vi "Cycling_No_DAQ_Tasks_All_3_PS.vi"() -> ()   [LabVIEW 2020]
uses:
  Desktop/Battery-Testing-Software - Shortcut.lnk/Drivers-IT-M3400/IT-M3400.lvlib
panel:
  in  "Number of Cycles 3":i32
  in  "Charge filepath 3":path
  in  "Discharge filepath 3":path
  in  "Batteryname 3":string
  in  "Starting Cycle 3":i32
  out "PS Visa Out 3":refnum<visa-resource-name>
  out "PS error out 3":errorcluster
  in  "Wait time 3":dbl
  in  "Discharge Current Setpoint 3":dbl format="%#.6g"
  in  "Charge Current Setpoint 3":dbl format="%#.6g"
  in  "Battery Type 3":enum16{"30Q", "40T"}(ring)
  in  "PS type 3":enum16{"NHR", "ITECH"}(ring)
  in  "PS error in 3":errorcluster caption="PS error in (no error)"
  in  "PS VISA in 3":refnum<visa-resource-name>
  in  "Number of Cycles 2":i32
  in  "Charge filepath 2":path
  in  "Discharge filepath 2":path
  in  "Batteryname 2":string
  in  "Starting Cycle 2":i32
  out "PS Visa Out 2":refnum<visa-resource-name>
  out "PS error out 2":errorcluster
  in  "Wait time 2":dbl
  in  "Discharge Current Setpoint 2":dbl format="%#.6g"
  in  "Charge Current Setpoint 2":dbl format="%#.6g"
  in  "Battery Type 2":enum16{"30Q", "40T"}(ring)
  in  "PS type 2":enum16{"NHR", "ITECH"}(ring)
  in  "PS error in 2":errorcluster caption="PS error in (no error)"
  in  "PS VISA in 2":refnum<visa-resource-name>
  in  "Number of Cycles":i32
  in  "Charge filepath":path
  in  "Discharge filepath":path
  in  "Batteryname":string
  in  "Starting Cycle":i32
  out "PS error out":errorcluster
  out "PS Visa Out":refnum<visa-resource-name>
  in  "Wait time":dbl
  in  "Discharge Current Setpoint":dbl format="%#.6g"
  in  "Charge Current Setpoint":dbl format="%#.6g"
  in  "Battery Type":enum16{"30Q", "40T"}(ring)
  in  "PS type":enum16{"NHR", "ITECH"}(ring)
  in  "PS error in":errorcluster caption="PS error in (no error)"
  in  "PS VISA in":refnum<visa-resource-name>
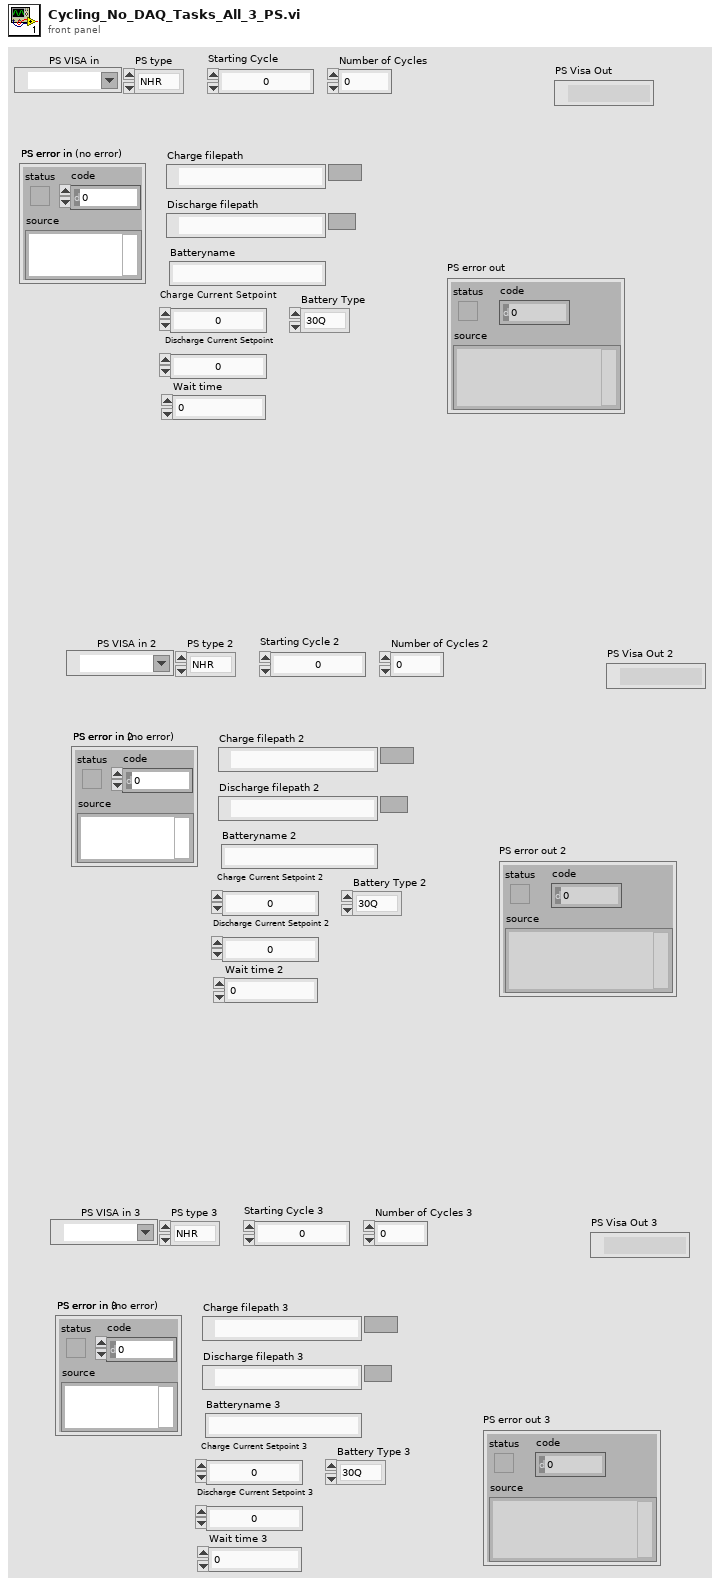
[diagram p1: front panel]
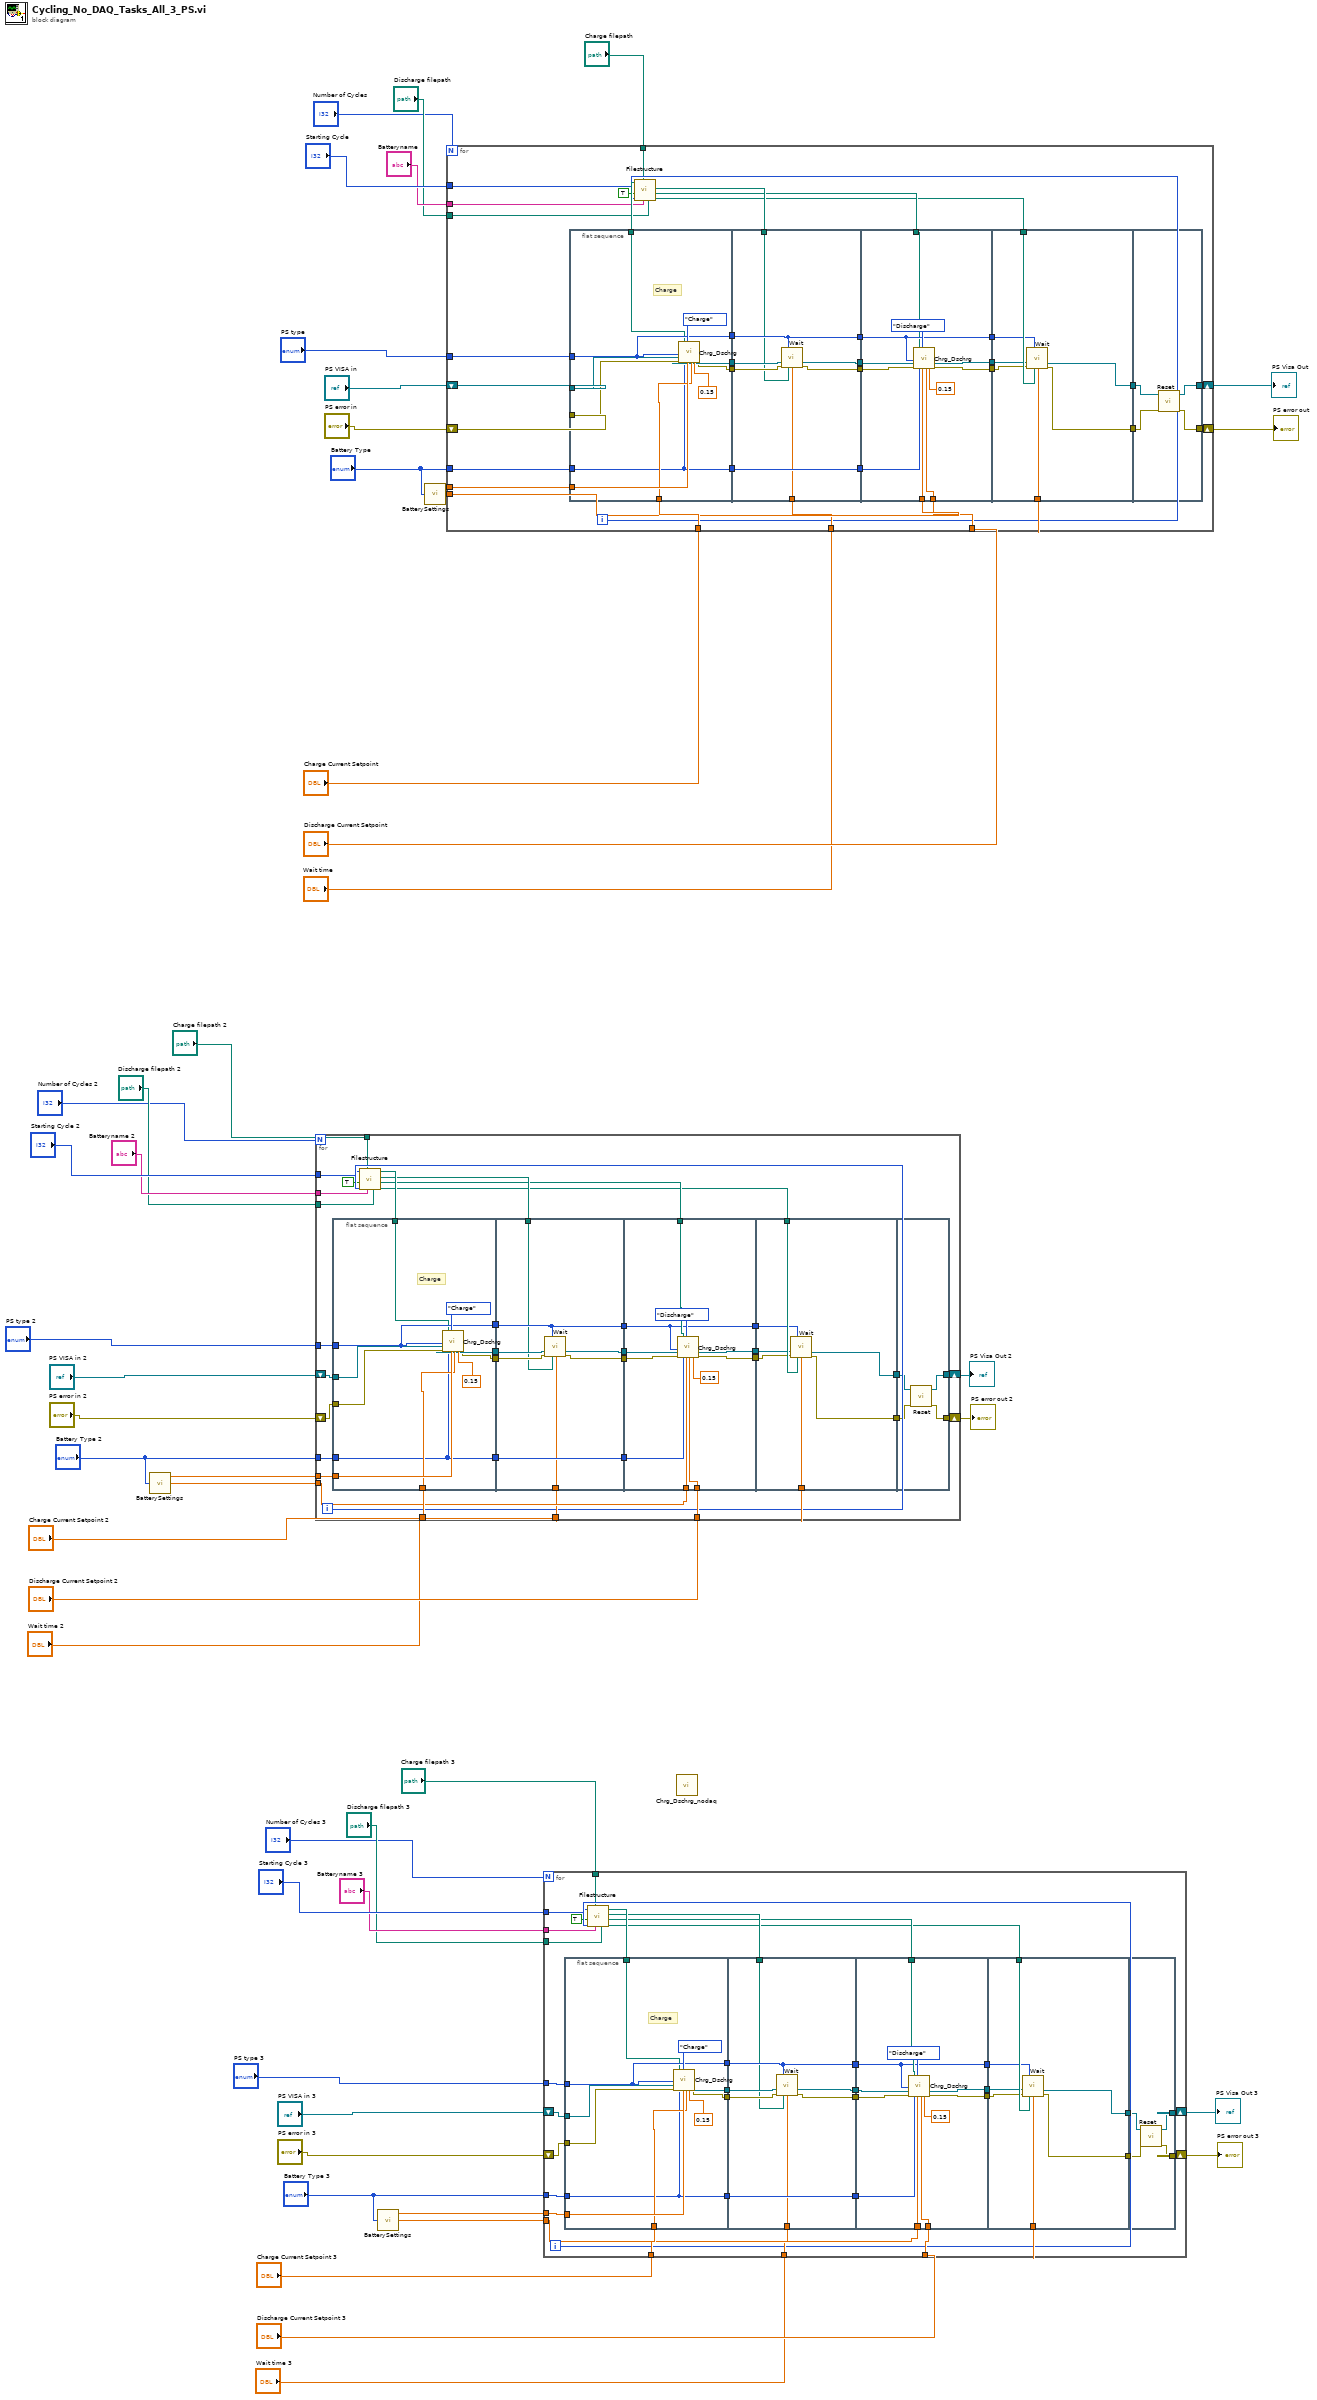
[diagram p0: block diagram]
diagram:
  n1 = call "BatterySettings.vi"("Battery Type"="Battery Type 2") -> ("Min Voltage (V)"=w26:dbl, "Max Voltage (V)"=w29:dbl)  [unwired: 2 in, 1 out]
  n2 = for {
    N: "Number of Cycles 2" -> [_]
    tunnel: "PS type 2" -> [w71]
    tunnel: w29 -> [w68]
    tunnel: "Battery Type 2" -> [w67]
    tunnel: "Charge Current Setpoint 2" -> [w66]
    tunnel: w26 -> [w65]
    tunnel: "Discharge Current Setpoint 2" -> [w64]
    tunnel: "Wait time 2" -> [w59]
    shift-right: [w57] -> w22
    shift-left: "PS VISA in 2" -> [w70]
    shift-right: [w58] -> w23
    shift-left: "PS error in 2" -> [w69]
    tunnel: "Starting Cycle 2" -> [w55]
    tunnel: "Batteryname 2" -> [w53]
    tunnel: "Discharge filepath 2" -> [w52]
    tunnel: "Charge filepath 2" -> [w51]
    i -> [w56]
    n3 = flat-sequence {
      tunnel: w71 -> [w85]
      tunnel: w70 -> [w93]
      tunnel: w69 -> [w92]
      tunnel: w67 -> [w84]
      tunnel: w68 -> [w89]
      tunnel: w66 -> [w88]
      tunnel: [w87] -> w82
      tunnel: [w86] -> w81
      tunnel: [w85] -> w80
      tunnel: [w84] -> w79
      tunnel: w63 -> [w83]
      tunnel: w82 -> [w101]
      tunnel: w81 -> [w100]
      tunnel: w80 -> [w97]
      tunnel: [w99] -> w78
      tunnel: [w98] -> w77
      tunnel: [w97] -> w76
      tunnel: w79 -> [w96]
      tunnel: [w96] -> w75
      tunnel: w62 -> [w95]
      tunnel: w59 -> [w94]
      tunnel: w78 -> [w112]
      tunnel: w77 -> [w111]
      tunnel: w76 -> [w102]
      tunnel: w75 -> [w110]
      tunnel: w65 -> [w109]
      tunnel: w64 -> [w108]
      tunnel: w61 -> [w105]
      tunnel: [w104] -> w74
      tunnel: [w103] -> w73
      tunnel: [w102] -> w72
      tunnel: w60 -> [w119]
      tunnel: w74 -> [w118]
      tunnel: w73 -> [w117]
      tunnel: w59 -> [w116]
      tunnel: w72 -> [w115]
      tunnel: [w114] -> w50
      tunnel: [w113] -> w49
      tunnel: [w122] -> w57
      tunnel: [w120] -> w58
      tunnel: w50 -> [w121]
      tunnel: w49 -> [w123]
      frame #0 {
        # "Charge"
        n4 = call "Chrg_Dschrg.vi"("PS type"=w85, "PS VISA in"=w93, "PS error in"=w92, "DischargeCyclePath"=w83, "Battery Type"=w84, "Charge/discharge"=enum8{"Charge", "Discharge"}."Charge", "Charge/Discharge Voltage Setpoint"=w89, "Current Setpoint"=w88, "Current Cutoff"=0.15) -> ("PS VIS resource name out"=w87:refnum<visa-resource-name>, "PS error out"=w86:errorcluster)  [unwired: 7 in, 2 out]
      }
      frame #1 {
        n5 = call "Wait.vi"("PS type"=w97, "PS VISA in"=w101, "PS error in"=w100, "Wait Filepath"=w95, "Wait time"=w94) -> ("PS Visa Out"=w99:refnum<visa-resource-name>, "PS error out"=w98:errorcluster)  [unwired: 7 in, 2 out]
      }
      frame #2 {
        n6 = call "Chrg_Dschrg.vi"("PS type"=w102, "PS VISA in"=w112, "PS error in"=w111, "DischargeCyclePath"=w105, "Battery Type"=w110, "Charge/discharge"=enum8{"Charge", "Discharge"}."Discharge", "Charge/Discharge Voltage Setpoint"=w109, "Current Setpoint"=w108, "Current Cutoff"=0.15) -> ("PS VIS resource name out"=w104:refnum<visa-resource-name>, "PS error out"=w103:errorcluster)  [unwired: 7 in, 2 out]
      }
      frame #3 {
        n7 = call "Wait.vi"("PS type"=w115, "PS VISA in"=w118, "PS error in"=w117, "Wait Filepath"=w119, "Wait time"=w116) -> ("PS Visa Out"=w113:refnum<visa-resource-name>, "PS error out"=w114:errorcluster)  [unwired: 7 in, 2 out]
      }
      frame #4 {
        n8 = call "Reset.vi"("error in"=w121, "VISA resource name"=w123) -> ("error out"=w120:errorcluster, "VISA resource name out"=w122:refnum<visa-resource-name>)  [unwired: 8 in]
      }
    }
    n9 = call "Filestructure.vi"("Discharge filepath"=w52, "Batteryname"=w53, "Charge filepath"=w51, "For loop i"=w56, "In for loop"=TRUE, "Starting Cycle"=w55) -> ("DischargeWaitPath"=w60:path, "DischargeCyclePath"=w61:path, "ChargeWaitPath"=w62:path, "ChargeCyclePath"=w63:path)  [unwired: 1 in, 1 out]
  }
  "PS error out 2" <- w23
  "PS Visa Out 2" <- w22
  n10 = call "BatterySettings.vi"("Battery Type"="Battery Type 3") -> ("Min Voltage (V)"=w10:dbl, "Max Voltage (V)"=w13:dbl)  [unwired: 2 in, 1 out]
  n11 = call "BatterySettings.vi"("Battery Type"="Battery Type") -> ("Min Voltage (V)"=w42:dbl, "Max Voltage (V)"=w45:dbl)  [unwired: 2 in, 1 out]
  n12 = for {
    N: "Number of Cycles" -> [_]
    tunnel: "PS type" -> [w146]
    tunnel: w45 -> [w143]
    tunnel: "Battery Type" -> [w142]
    tunnel: "Charge Current Setpoint" -> [w141]
    tunnel: w42 -> [w140]
    tunnel: "Discharge Current Setpoint" -> [w139]
    tunnel: "Wait time" -> [w134]
    shift-right: [w132] -> w38
    shift-left: "PS VISA in" -> [w145]
    shift-right: [w133] -> w39
    shift-left: "PS error in" -> [w144]
    tunnel: "Starting Cycle" -> [w130]
    tunnel: "Batteryname" -> [w128]
    tunnel: "Discharge filepath" -> [w127]
    tunnel: "Charge filepath" -> [w126]
    i -> [w131]
    n13 = flat-sequence {
      tunnel: w146 -> [w160]
      tunnel: w145 -> [w168]
      tunnel: w144 -> [w167]
      tunnel: w142 -> [w159]
      tunnel: w143 -> [w164]
      tunnel: w141 -> [w163]
      tunnel: [w162] -> w157
      tunnel: [w161] -> w156
      tunnel: [w160] -> w155
      tunnel: [w159] -> w154
      tunnel: w138 -> [w158]
      tunnel: w157 -> [w176]
      tunnel: w156 -> [w175]
      tunnel: w155 -> [w172]
      tunnel: [w174] -> w153
      tunnel: [w173] -> w152
      tunnel: [w172] -> w151
      tunnel: w154 -> [w171]
      tunnel: [w171] -> w150
      tunnel: w137 -> [w170]
      tunnel: w134 -> [w169]
      tunnel: w153 -> [w187]
      tunnel: w152 -> [w186]
      tunnel: w151 -> [w178]
      tunnel: w150 -> [w185]
      tunnel: w140 -> [w184]
      tunnel: w139 -> [w183]
      tunnel: w136 -> [w177]
      tunnel: [w180] -> w149
      tunnel: [w179] -> w148
      tunnel: [w178] -> w147
      tunnel: w135 -> [w194]
      tunnel: w149 -> [w193]
      tunnel: w148 -> [w192]
      tunnel: w134 -> [w191]
      tunnel: w147 -> [w190]
      tunnel: [w189] -> w125
      tunnel: [w188] -> w124
      tunnel: [w197] -> w132
      tunnel: [w195] -> w133
      tunnel: w125 -> [w196]
      tunnel: w124 -> [w198]
      frame #0 {
        # "Charge"
        n14 = call "Chrg_Dschrg.vi"("PS type"=w160, "PS VISA in"=w168, "PS error in"=w167, "DischargeCyclePath"=w158, "Battery Type"=w159, "Charge/discharge"=enum8{"Charge", "Discharge"}."Charge", "Charge/Discharge Voltage Setpoint"=w164, "Current Setpoint"=w163, "Current Cutoff"=0.15) -> ("PS VIS resource name out"=w162:refnum<visa-resource-name>, "PS error out"=w161:errorcluster)  [unwired: 7 in, 2 out]
      }
      frame #1 {
        n15 = call "Wait.vi"("PS type"=w172, "PS VISA in"=w176, "PS error in"=w175, "Wait Filepath"=w170, "Wait time"=w169) -> ("PS Visa Out"=w174:refnum<visa-resource-name>, "PS error out"=w173:errorcluster)  [unwired: 7 in, 2 out]
      }
      frame #2 {
        n16 = call "Chrg_Dschrg.vi"("PS type"=w178, "PS VISA in"=w187, "PS error in"=w186, "DischargeCyclePath"=w177, "Battery Type"=w185, "Charge/discharge"=enum8{"Charge", "Discharge"}."Discharge", "Charge/Discharge Voltage Setpoint"=w184, "Current Setpoint"=w183, "Current Cutoff"=0.15) -> ("PS VIS resource name out"=w180:refnum<visa-resource-name>, "PS error out"=w179:errorcluster)  [unwired: 7 in, 2 out]
      }
      frame #3 {
        n17 = call "Wait.vi"("PS type"=w190, "PS VISA in"=w193, "PS error in"=w192, "Wait Filepath"=w194, "Wait time"=w191) -> ("PS Visa Out"=w188:refnum<visa-resource-name>, "PS error out"=w189:errorcluster)  [unwired: 7 in, 2 out]
      }
      frame #4 {
        n18 = call "Reset.vi"("error in"=w196, "VISA resource name"=w198) -> ("error out"=w195:errorcluster, "VISA resource name out"=w197:refnum<visa-resource-name>)  [unwired: 8 in]
      }
    }
    n19 = call "Filestructure.vi"("Discharge filepath"=w127, "Batteryname"=w128, "Charge filepath"=w126, "For loop i"=w131, "In for loop"=TRUE, "Starting Cycle"=w130) -> ("DischargeWaitPath"=w135:path, "DischargeCyclePath"=w136:path, "ChargeWaitPath"=w137:path, "ChargeCyclePath"=w138:path)  [unwired: 1 in, 1 out]
  }
  "PS error out" <- w39
  "PS Visa Out" <- w38
  n20 = for {
    N: "Number of Cycles 3" -> [_]
    tunnel: "PS type 3" -> [w221]
    tunnel: w13 -> [w218]
    tunnel: "Battery Type 3" -> [w217]
    tunnel: "Charge Current Setpoint 3" -> [w216]
    tunnel: w10 -> [w215]
    tunnel: "Discharge Current Setpoint 3" -> [w214]
    tunnel: "Wait time 3" -> [w209]
    shift-right: [w207] -> w6
    shift-left: "PS VISA in 3" -> [w220]
    shift-right: [w208] -> w7
    shift-left: "PS error in 3" -> [w219]
    tunnel: "Starting Cycle 3" -> [w205]
    tunnel: "Batteryname 3" -> [w203]
    tunnel: "Discharge filepath 3" -> [w202]
    tunnel: "Charge filepath 3" -> [w201]
    i -> [w206]
    n21 = flat-sequence {
      tunnel: w221 -> [w235]
      tunnel: w220 -> [w243]
      tunnel: w219 -> [w242]
      tunnel: w217 -> [w234]
      tunnel: w218 -> [w239]
      tunnel: w216 -> [w238]
      tunnel: [w237] -> w232
      tunnel: [w236] -> w231
      tunnel: [w235] -> w230
      tunnel: [w234] -> w229
      tunnel: w213 -> [w233]
      tunnel: w232 -> [w251]
      tunnel: w231 -> [w250]
      tunnel: w230 -> [w247]
      tunnel: [w249] -> w228
      tunnel: [w248] -> w227
      tunnel: [w247] -> w226
      tunnel: w229 -> [w246]
      tunnel: [w246] -> w225
      tunnel: w212 -> [w245]
      tunnel: w209 -> [w244]
      tunnel: w228 -> [w262]
      tunnel: w227 -> [w261]
      tunnel: w226 -> [w252]
      tunnel: w225 -> [w260]
      tunnel: w215 -> [w259]
      tunnel: w214 -> [w258]
      tunnel: w211 -> [w255]
      tunnel: [w254] -> w224
      tunnel: [w253] -> w223
      tunnel: [w252] -> w222
      tunnel: w210 -> [w269]
      tunnel: w224 -> [w268]
      tunnel: w223 -> [w267]
      tunnel: w209 -> [w266]
      tunnel: w222 -> [w265]
      tunnel: [w264] -> w200
      tunnel: [w263] -> w199
      tunnel: [w272] -> w207
      tunnel: [w270] -> w208
      tunnel: w200 -> [w271]
      tunnel: w199 -> [w273]
      frame #0 {
        # "Charge"
        n22 = call "Chrg_Dschrg.vi"("PS type"=w235, "PS VISA in"=w243, "PS error in"=w242, "DischargeCyclePath"=w233, "Battery Type"=w234, "Charge/discharge"=enum8{"Charge", "Discharge"}."Charge", "Charge/Discharge Voltage Setpoint"=w239, "Current Setpoint"=w238, "Current Cutoff"=0.15) -> ("PS VIS resource name out"=w237:refnum<visa-resource-name>, "PS error out"=w236:errorcluster)  [unwired: 7 in, 2 out]
      }
      frame #1 {
        n23 = call "Wait.vi"("PS type"=w247, "PS VISA in"=w251, "PS error in"=w250, "Wait Filepath"=w245, "Wait time"=w244) -> ("PS Visa Out"=w249:refnum<visa-resource-name>, "PS error out"=w248:errorcluster)  [unwired: 7 in, 2 out]
      }
      frame #2 {
        n24 = call "Chrg_Dschrg.vi"("PS type"=w252, "PS VISA in"=w262, "PS error in"=w261, "DischargeCyclePath"=w255, "Battery Type"=w260, "Charge/discharge"=enum8{"Charge", "Discharge"}."Discharge", "Charge/Discharge Voltage Setpoint"=w259, "Current Setpoint"=w258, "Current Cutoff"=0.15) -> ("PS VIS resource name out"=w254:refnum<visa-resource-name>, "PS error out"=w253:errorcluster)  [unwired: 7 in, 2 out]
      }
      frame #3 {
        n25 = call "Wait.vi"("PS type"=w265, "PS VISA in"=w268, "PS error in"=w267, "Wait Filepath"=w269, "Wait time"=w266) -> ("PS Visa Out"=w263:refnum<visa-resource-name>, "PS error out"=w264:errorcluster)  [unwired: 7 in, 2 out]
      }
      frame #4 {
        n26 = call "Reset.vi"("error in"=w271, "VISA resource name"=w273) -> ("error out"=w270:errorcluster, "VISA resource name out"=w272:refnum<visa-resource-name>)  [unwired: 8 in]
      }
    }
    n27 = call "Filestructure.vi"("Discharge filepath"=w202, "Batteryname"=w203, "Charge filepath"=w201, "For loop i"=w206, "In for loop"=TRUE, "Starting Cycle"=w205) -> ("DischargeWaitPath"=w210:path, "DischargeCyclePath"=w211:path, "ChargeWaitPath"=w212:path, "ChargeCyclePath"=w213:path)  [unwired: 1 in, 1 out]
  }
  "PS error out 3" <- w7
  "PS Visa Out 3" <- w6
  n28 = call "Chrg_Dschrg_nodaq.vi"() -> ()  [unwired: 18 in, 2 out]
